vi "Set DAQ data API.vi"(7 "Config":T1 {"Config"."Input Config" items=["default"=-1, "RSE"=10083, "NRSE"=10078, "Differential"=10106, "Pseudodifferential"=12529]}, 8 "Error In":errorcluster) -> (0 "Error Out":errorcluster)   [LabVIEW 2017, in "UI.lvlib"]
uses:
  UI.lvlib
  DAQ/Controls/Params.ctl
  DAQ/Controls/DAQ Config.ctl
  DAQ/Controls/DAQ Indicators.ctl
  System Control/CTLs/Test Type.ctl
  Controls/Command Data [cluster].ctl
  Controls/Commands [enum].ctl
  Events/Events.lvlib
  DAQ/DAQ.lvlib
  System Control/Main controller.lvlib
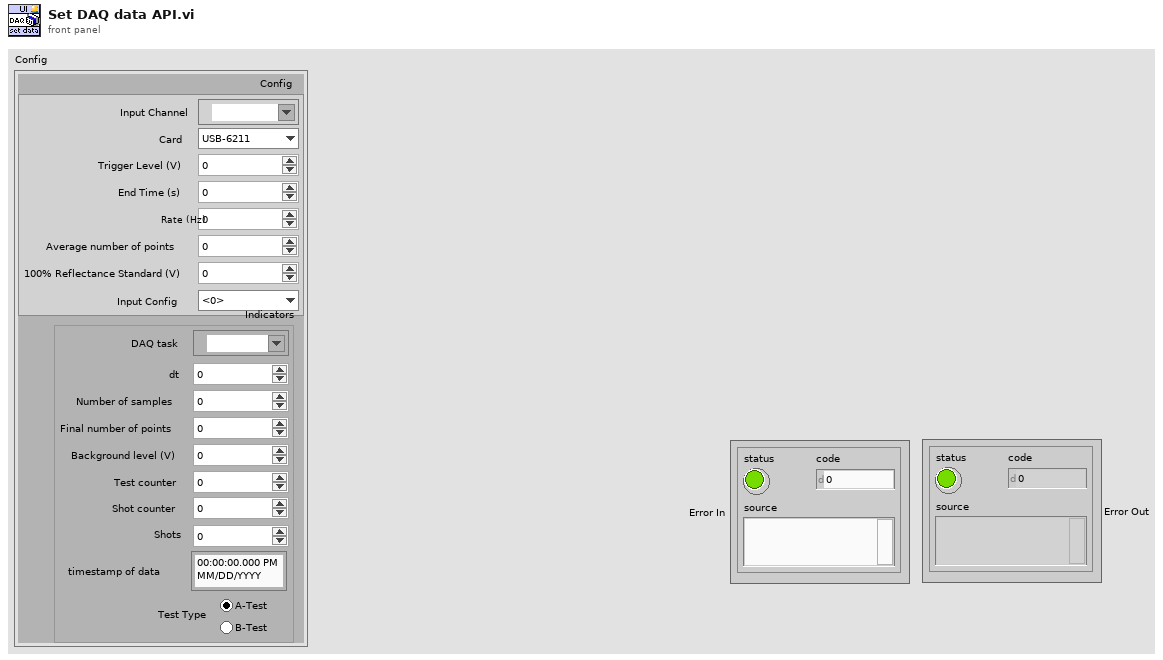
[diagram p1: front panel]
types:
  T1 = typedef "DAQ.lvlib/Params.ctl" = cluster{"Data":cluster{"Live":waveform(dbl), "Accumulated":waveform(dbl), "Averaged":waveform(dbl), "data array":dbl[], "live time array":dbl[], "Live (decimated)":waveform(dbl)}, "Config":T2, "Indicators":T3}
  T2 = typedef "DAQ.lvlib/DAQ Config.ctl" = cluster{"Input Config":i32, "Card":enum16{"USB-6211", "USB-6251", "USB-6361"}, "100% Reflectance Standard (V)":dbl, "Input Channel":tag, "Average number of points":dbl, "Trigger Level (V)":dbl, "Rate (Hz)":i32, "End Time (s)":dbl}
  T3 = typedef "DAQ.lvlib/DAQ Indicators.ctl" = cluster{"Final number of points":dbl, "Number of samples":dbl, "dt":dbl, "Shots":i32, "Shot counter":i32, "Test counter":i32, "Background level (V)":dbl, "DAQ task":refnum<k21>, "timestamp of data":timestamp, "Test Type":T4}
  T4 = typedef "Main controller.lvlib/Test Type.ctl" = enum32{"A-Test", "B-Test"}
  T5 = typedef "UI.lvlib/Command Data [cluster].ctl" = cluster{"Command":T6, "Data":variant}
  T6 = typedef "UI.lvlib/Commands [enum].ctl" = enum16{"Start", "Update", "Acquisition Complete", "Stop", "Set DAQ data", "Set Scope data", "Set processing data", "Clear Graphs"}
  T7 = typedef "Events.lvlib/Refs [cluster].ctl" = cluster{"Exit":refnum<user-event>, "Controller":refnum<user-event>, "System Error":refnum<user-event>, "UI":refnum<user-event>, "Example Module":refnum<user-event>, "Shutter":refnum<user-event>, "Monochromator":refnum<user-event>, "DAQ":refnum<user-event>, "Scope":refnum<user-event>, "Processing":refnum<user-event>, "File IO":refnum<user-event>, "Colour wheel":refnum<user-event>}
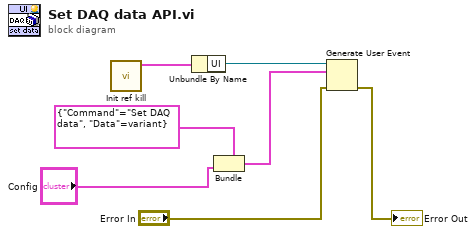
[diagram p0: block diagram]
diagram:
  n1 = call "Init ref kill.vi"() -> ("Messages"=w7:T7)  [unwired: 10 in, 1 out]
  n2 = Unbundle By Name(w7) -> ("UI"=w6:refnum<user-event>)
  n3 = Bundle(cluster=T5 {"Command"=enum."Set DAQ data", "Data"=variant} ("event data"), "Data"="Config") -> (w2:T5)  [unwired: 1 in]
  n4 = Generate User Event(user event=w6, event data cluster=w2, error in="Error In") -> (error out=→"Error Out":errorcluster)  [unwired: 1 in, 1 out]
